vi "Include Limit in Compare String.vi"(11 "include limit in compare":bool) -> (3 "compare":string)   [LabVIEW 2020, in "Static Errors.lvlib"]
uses:
  Static Errors.lvlib
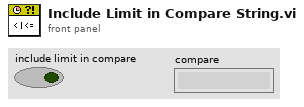
[diagram p1: front panel]
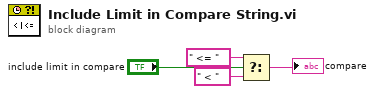
[diagram p0: block diagram]
diagram:
  n1 = Select(t=" <= ", s="include limit in compare", f=" < ") -> (s? t:f=→"compare":string)
